vi "Sort Panels.vi"(8 "error in (no error)":errorcluster, 10 "Sort VI":T1, 11 "ArrayManager in":refnum<class "ArrayManager.lvclass">) -> (0 "error out":errorcluster, 3 "ArrayManager out":refnum<class "ArrayManager.lvclass">)   [LabVIEW 2020, in "OOPanel.lvlib" / "ArrayManager.lvclass"]
uses:
  ArrayManager.lvclass
  Sort VI Type.ctl
  Panel/Panel.lvclass
  ArrayManager.lvclass/ArrayManager.ctl
  ArrayPanel/ArrayPanel.lvclass
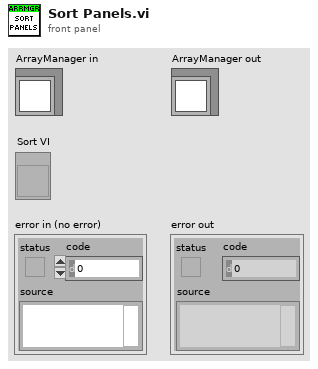
[diagram p1: front panel]
types:
  T1 = typedef "OOPanel.lvlib/ArrayManager.lvclass/Sort VI Type.ctl" = refnum<vi>
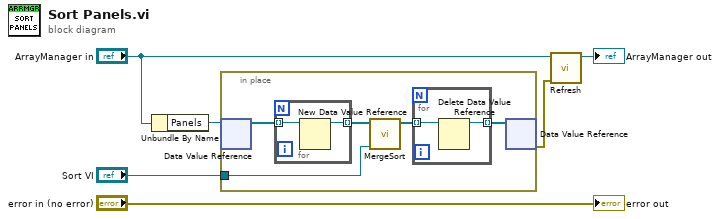
[diagram p0: block diagram]
diagram:
  n1 = Unbundle By Name("ArrayManager in") -> ("Panels"=w5:refnum<data-value>)
  n2 = in-place {
    in-place-border: "Sort VI" -> [w8]
    n3 = in-place-dvr #1(w5) -> (w11:refnum<class "ArrayPanel.lvclass">[])  [unwired: 1 out]
    n4 = for {
      tunnel: w11 -> [w13] mode=indexing
      tunnel: [w12] -> w9 mode=indexing
      n5 = New Data Value Reference(data value=w13) -> (data value reference=w12:refnum<data-value>)  [unwired: 1 in, 1 out]
    }
    n6 = call "MergeSort.vi"("Sort VI"=w8, "ArrayPanelRefs"=w9) -> ("Sorted ArrayPanelRefs"=w7:refnum<data-value>[])  [unwired: 9 in]
    n7 = for {
      tunnel: [w15] -> w10 mode=indexing
      tunnel: w7 -> [w14] mode=indexing
      n8 = Delete Data Value Reference(data value reference=w14) -> (data value=w15:refnum<class "ArrayPanel.lvclass">)  [unwired: 1 in, 1 out]
    }
    n9 = in-place-dvr #1(w10) -> (w1:errorcluster)  [unwired: 1 out]
  }
  n10 = call "Refresh.vi"("error in (no error)"=w1, "ArrayManager in"="ArrayManager in") -> ("ArrayManager out"=→"ArrayManager out":refnum<class "ArrayManager.lvclass">)  [unwired: 8 in, 1 out]
  "error out" <- "error in (no error)"
